vi "zmq_endpoint_split.vi"(4 "error in":errorcluster, 7 "endpoint":string) -> (0 "error out":errorcluster, 1 "port":u16, 2 "address":string="127.0.0.1", 3 "protocol":T1)   [LabVIEW 2020, in "zeromq.lvlib"]
doc: "Convenience function to split an endpoint string into its parts.\n\nProduces EINVAL if the given string is not a valid endpoint, and EPROTONOSUPPORT if the protocol is not supported."
uses:
  zeromq.lvlib
  endpoint_proto.ctl
  Match Regular Expression.xnode
panel:
  # "ØMQ"
  # "labview"
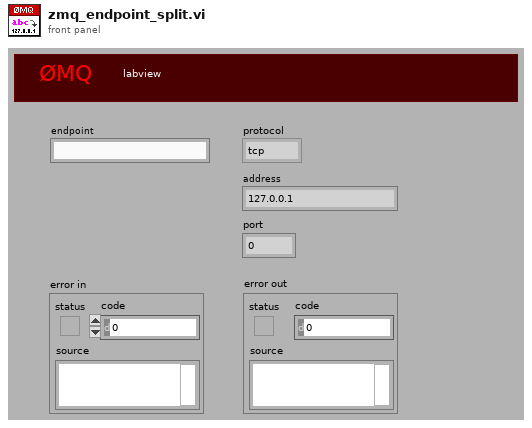
[diagram p1: front panel]
types:
  T1 = typedef "zeromq.lvlib/endpoint_proto.ctl" = enum16{"tcp", "inproc"}
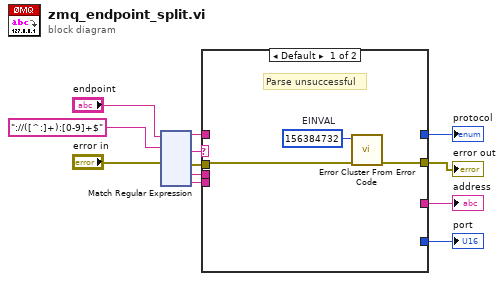
[diagram p0: block diagram]
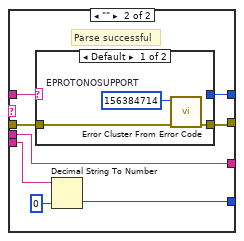
[diagram p2: hidden frame]
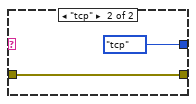
[diagram p3: hidden frame]
diagram:
  n1 = xnode "Match Regular Expression"("input string"="endpoint", "regular expression"="://([^:]+):[0-9]+$", "error in"="error in") -> ("before match"=w9:string, "after match"=w4:string, "error out"=w5:errorcluster, "submatch 1"=w2:string, "submatch 2"=w7:string)  [unwired: 3 in, 2 out]
  n2 = case shown="Default" w4 {
    tunnel: w9 -> [_ w23]
    tunnel: [_ w22] -> w8
    tunnel: w7 -> [_ w21]
    tunnel: [_ w20] -> w6
    tunnel: w5 -> [w15 w18]
    tunnel: [w14 w17] -> w3
    tunnel: w2 -> [_ w16]
    tunnel: [_ w16] -> w1
    frame Default {
      w13 = 156384732  # EINVAL
      # "Parse unsuccessful"
      n3 = call "Error Cluster From Error Code.vi"("error in (no error)"=w15, "error code (0)"=w13) -> ("error out"=w14:errorcluster)  [unwired: 7 in]
    }
    frame "" {
      # "Parse successful"
      n4 = case shown="Default" w23 {
        tunnel: [_ enum16{"tcp", "inproc"}."tcp" ("protocol")] -> w22
        tunnel: w18 -> [w25 w27]
        tunnel: [w26 w27] -> w17
        frame Default {
          w24 = 156384714  # EPROTONOSUPPORT
          n5 = call "Error Cluster From Error Code.vi"("error in (no error)"=w25, "error code (0)"=w24) -> ("error out"=w26:errorcluster)  [unwired: 7 in]
        }
        frame "tcp" {
        }
      }
      n6 = Decimal String To Number(string=w21, default (0L)=u16 0 ("default (0 I32)")) -> (number=w20:u16)  [unwired: 1 in, 1 out]
    }
  }
  "address" <- w1
  "error out" <- w3
  "protocol" <- w8
  "port" <- w6
